vi "DDS Inits.vi"() -> (0 "error out":errorcluster, 2 "DDS Reader out":refnum<class "DDS Reader.lvclass">, 3 "DDS Writer out":refnum<class "DDS Writer.lvclass">)   [LabVIEW 2018]
uses:
  <vilib>/ORNL/CSEISMIC DDS/DDS Writer/DDS Writer.lvclass
  C:/Program Files (x86)/National Instruments/LabVIEW 2018/vi.lib/ORNL/CSEISMIC DDS/CSEISMIC DDS Base/CSEISMIC DDS.lvclass
  <vilib>/ORNL/CSEISMIC DDS/DDS Reader/DDS Reader.lvclass
  <vilib>/ORNL/CSEISMIC DDS/CSEISMIC DDS Base/CSEISMIC DDS.lvclass/CSEISMIC DDS.ctl
  <vilib>/ORNL/CSEISMIC DDS/CSEISMIC DDS Base/Accessors/Write DDS Reference.vi
  <vilib>/ORNL/CSEISMIC DDS/CSEISMIC DDS Base/Error Handler.vi
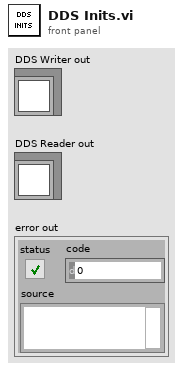
[diagram p1: front panel]
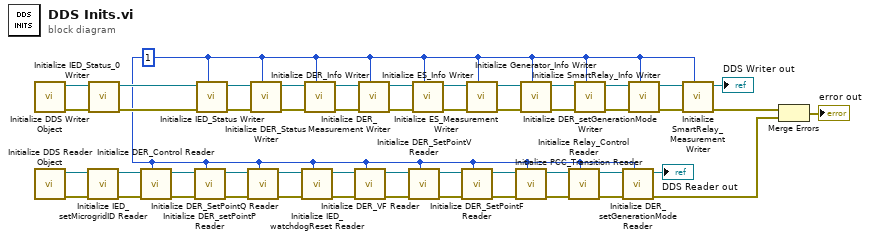
[diagram p0: block diagram]
diagram:
  w1 = u32 1 ("MicrogridID")
  n1 = call <vilib>:"Initialize DDS Writer Object.vi"() -> ("error out"=w50:errorcluster, "DDS Writer out"=w49:refnum<class "DDS Writer.lvclass">)  [unwired: 10 in]
  n2 = call <vilib>:"Initialize DDS Reader Object.vi"() -> ("error out"=w48:errorcluster, "DDS Reader out"=w47:refnum<class "DDS Reader.lvclass">)  [unwired: 10 in]
  n3 = call <vilib>:"Initialize IED_setMicrogridID Reader.vi"("error in"=w48, "DDS Reader in"=w47) -> ("error out"=w34:errorcluster, "DDS Reader out"=w33:refnum<class "DDS Reader.lvclass">)  [unwired: 8 in]
  n4 = call <vilib>:"Initialize IED_Status_0 Writer.vi"("error in"=w50, "DDS Writer in"=w49) -> ("error out"=w32:errorcluster, "DDS Writer out"=w31:refnum<class "DDS Writer.lvclass">)  [unwired: 8 in]
  n5 = call <vilib>:"Initialize DER_Control Reader.vi"("MicrogridID"=w1, "error in"=w34, "DDS Reader in"=w33) -> ("error out"=w43:errorcluster, "DDS Reader out"=w37:refnum<class "DDS Reader.lvclass">)  [unwired: 7 in]
  n6 = call <vilib>:"Initialize DER_setPointP Reader.vi"("MicrogridID"=w1, "error in"=w43, "DDS Reader in"=w37) -> ("error out"=w42:errorcluster, "DDS Reader out"=w36:refnum<class "DDS Reader.lvclass">)  [unwired: 7 in]
  n7 = call <vilib>:"Initialize IED_Status Writer.vi"("MicrogridID"=w1, "error in"=w32, "DDS Writer in"=w31) -> ("error out"=w46:errorcluster, "DDS Writer out"=w40:refnum<class "DDS Writer.lvclass">)  [unwired: 7 in]
  n8 = call <vilib>:"Initialize DER_SetPointQ Reader.vi"("MicrogridID"=w1, "error in"=w42, "DDS Reader in"=w36) -> ("error out"=w41:errorcluster, "DDS Reader out"=w35:refnum<class "DDS Reader.lvclass">)  [unwired: 7 in]
  n9 = call <vilib>:"Initialize DER_Status Writer.vi"("MicrogridID"=w1, "error in"=w46, "DDS Writer in"=w40) -> ("error out"=w45:errorcluster, "DDS Writer out"=w39:refnum<class "DDS Writer.lvclass">)  [unwired: 7 in]
  n10 = call <vilib>:"Initialize IED_watchdogReset Reader.vi"("MicrogridID"=w1, "error in"=w41, "DDS Reader in"=w35) -> ("error out"=w27:errorcluster, "DDS Reader out"=w26:refnum<class "DDS Reader.lvclass">)  [unwired: 7 in]
  n11 = call <vilib>:"Initialize DER_Info Writer.vi"("MicrogridID"=w1, "error in"=w45, "DDS Writer in"=w39) -> ("error out"=w44:errorcluster, "DDS Writer out"=w38:refnum<class "DDS Writer.lvclass">)  [unwired: 7 in]
  n12 = call <vilib>:"Initialize DER_VF Reader.vi"("MicrogridID"=w1, "error in"=w27, "DDS Reader in"=w26) -> ("error out"=w28:errorcluster, "DDS Reader out"=w25:refnum<class "DDS Reader.lvclass">)  [unwired: 7 in]
  n13 = call <vilib>:"Initialize DER_Measurement Writer.vi"("MicrogridID"=w1, "error in"=w44, "DDS Writer in"=w38) -> ("error out"=w6:errorcluster, "DDS Writer"=w7:refnum<class "DDS Writer.lvclass">)  [unwired: 7 in]
  n14 = call <vilib>:"Initialize DER_SetPointV Reader.vi"("MicrogridID"=w1, "error in"=w28, "DDS Reader in"=w25) -> ("error out"=w3:errorcluster, "DDS Reader out"=w5:refnum<class "DDS Reader.lvclass">)  [unwired: 7 in]
  n15 = call <vilib>:"Initialize ES_Info Writer.vi"("MicrogridID"=w1, "error in"=w6, "DDS Writer in"=w7) -> ("error out"=w30:errorcluster, "DDS Writer out"=w29:refnum<class "DDS Writer.lvclass">)  [unwired: 7 in]
  n16 = call <vilib>:"Initialize DER_SetPointF Reader.vi"("MicrogridID"=w1, "error in"=w3, "DDS Reader in"=w5) -> ("error out"=w2:errorcluster, "DDS Reader out"=w4:refnum<class "DDS Reader.lvclass">)  [unwired: 7 in]
  n17 = call <vilib>:"Initialize ES_Measurement Writer.vi"("MicrogridID"=w1, "error in"=w30, "DDS Writer in"=w29) -> ("error out"=w24:errorcluster, "DDS Writer out"=w23:refnum<class "DDS Writer.lvclass">)  [unwired: 7 in]
  n18 = call <vilib>:"Initialize PCC_Transition Reader.vi"("MicrogridID"=w1, "error in"=w2, "DDS Reader in"=w4) -> ("error out"=w16:errorcluster, "DDS Reader out"=w13:refnum<class "DDS Reader.lvclass">)  [unwired: 7 in]
  n19 = call <vilib>:"Initialize Generator_Info Writer.vi"("MicrogridID"=w1, "error in"=w24, "DDS Writer in"=w23) -> ("error out"=w17:errorcluster, "DDS Writer out"=w20:refnum<class "DDS Writer.lvclass">)  [unwired: 7 in]
  n20 = call <vilib>:"Initialize Relay_Control Reader.vi"("MicrogridID"=w1, "error in"=w16, "DDS Reader in"=w13) -> ("error out"=w15:errorcluster, "DDS Reader out"=w14:refnum<class "DDS Reader.lvclass">)  [unwired: 7 in]
  n21 = call <vilib>:"Initialize DER_setGenerationMode Writer.vi"("MicrogridID"=w1, "error in"=w17, "DDS Writer in"=w20) -> ("error out"=w18:errorcluster, "DDS Writer out"=w19:refnum<class "DDS Writer.lvclass">)  [unwired: 7 in]
  n22 = call <vilib>:"Initialize DER_setGenerationMode Reader.vi"("MicrogridID"=w1, "error in"=w15, "DDS Reader in"=w14) -> ("error out"=w11:errorcluster, "DDS Reader out"=→"DDS Reader out":refnum<class "DDS Reader.lvclass">)  [unwired: 7 in]
  n23 = call <vilib>:"Initialize SmartRelay_Info Writer.vi"("MicrogridID"=w1, "error in"=w18, "DDS Writer in"=w19) -> ("error out"=w21:errorcluster, "DDS Writer out"=w22:refnum<class "DDS Writer.lvclass">)  [unwired: 7 in]
  n24 = call <vilib>:"Initialize SmartRelay_Measurement Writer.vi"("MicrogridID"=w1, "error in"=w21, "DDS Writer in"=w22) -> ("error out"=w12:errorcluster, "DDS Writer out"=→"DDS Writer out":refnum<class "DDS Writer.lvclass">)  [unwired: 7 in]
  n25 = Merge Errors(w12, w11) -> (→"error out":errorcluster)
